vi "Initialize.vi"(8 "error in (no error)":errorcluster, 11 "AF Trace Queue in":refnum<class "AF Trace Queue.lvclass">) -> (0 "error out":errorcluster, 3 "AF Trace Queue out":refnum<class "AF Trace Queue.lvclass">)   [LabVIEW 2020, in "AF Trace Queue.lvclass"]
uses:
  AF Trace Queue.lvclass
  AF Trace Queue.lvclass/AF Trace Queue.ctl
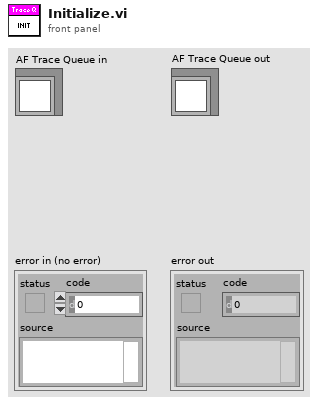
[diagram p1: front panel]
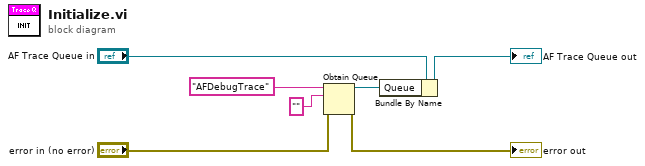
[diagram p0: block diagram]
diagram:
  n1 = Obtain Queue(name (unnamed)="AFDebugTrace" ("Name"), element data type="", error in (no error)="error in (no error)") -> (queue out=w5:refnum<queue>, error out=→"error out":errorcluster)  [unwired: 2 in, 1 out]
  n2 = Bundle By Name(cluster="AF Trace Queue in", "Queue"=w5) -> (→"AF Trace Queue out":refnum<class "AF Trace Queue.lvclass">)
